vi "Constants.vi"() -> ()   [LabVIEW 2015, in "RT Datalogger Shared.lvlib"]
doc: "Use this Global VI to access the GUIDs assigned to the page resources of the Custom Device."
uses:
  RT Datalogger Shared.lvlib
panel:
  in  "Tab Control":enum32{"GUIDS", "Constants", "Properties"}(tab)
  in  "RT Datalogger":string="a9b96f72-7fd4-4876-9d48-2a66e7c09004"
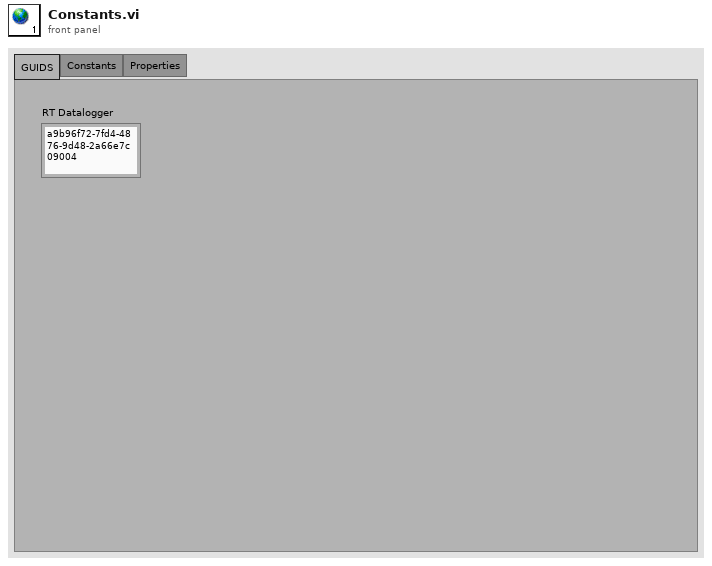
[diagram p1: front panel]
diagram:
